vi "BuildPlotsOneGraph.vi"(6 "Legend":string[](array[string]), 7 "Desired Legends":string[](array[string]), 8 "PlotArray":cluster{dbl[], dbl[]}[](array[cluster]), 9 "Plot Legends":string[](array[string]), 10 "Plotstyles":T1[](array[typedef]) {"LineType" min=1 max=6 step=1; "LineWidth" min=1 max=6 step=1; "PointSize" min=0 step=0.1}, 11 "PlotCommand":string) -> (0 "Yspan":dbl, 1 "Xspan":dbl, 3 "String out":string, 4 "Y array":dbl[](array[numeric]), 5 "X array":dbl[](array[numeric]))   [LabVIEW 2012]
uses:
  plotstyle.ctl
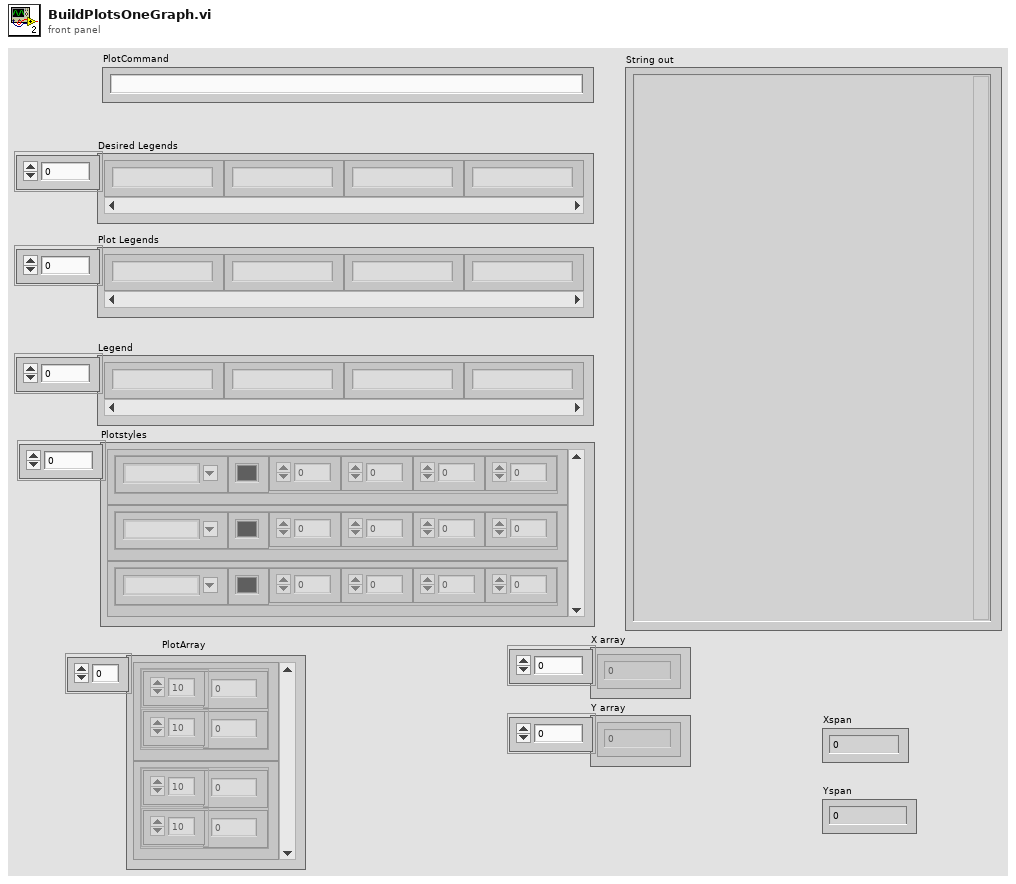
[diagram p1: front panel]
types:
  T1 = typedef "plotstyle.ctl" = cluster{"Style":string, "Color":u32, "PointType":i32, "PointSize":sgl, "LineWidth":sgl, "LineType":u8}
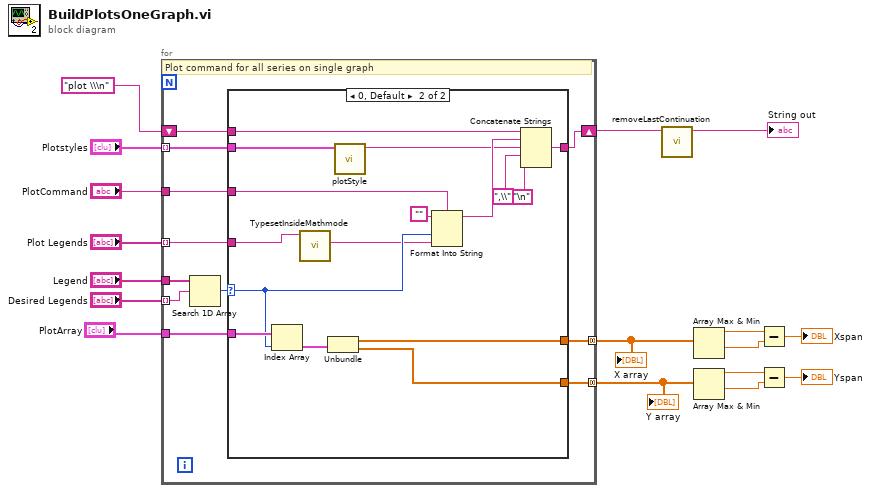
[diagram p0: block diagram]
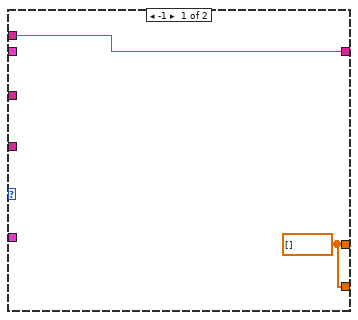
[diagram p2: hidden frame]
diagram:
  n1 = for {
    tunnel: "Plotstyles" -> [w28] mode=indexing
    tunnel: "Plot Legends" -> [w25] mode=indexing
    shift-right: [w26] -> w15
    shift-left: "plot \\\n" -> [w27]
    tunnel: "Desired Legends" -> [w23] mode=indexing
    tunnel: "Legend" -> [w24]
    tunnel: "PlotCommand" -> [w21]
    tunnel: "PlotArray" -> [w20]
    tunnel: [w19] -> w6 mode=concatenating
    tunnel: [w18] -> w3 mode=concatenating
    # "Plot command for all series on single graph"
    n2 = Search 1D Array(1D array=w24, element=w23) -> (index of element=w22:i32)  [unwired: 1 in]
    n3 = case shown="0, Default" w22 {
      selector: w22 -> [_ w36]
      tunnel: w28 -> [_ w45]
      tunnel: w27 -> [w30 w40]
      tunnel: [w30 w39] -> w26
      tunnel: w25 -> [_ w32]
      tunnel: w21 -> [_ w38]
      tunnel: w20 -> [_ w37]
      tunnel: [w29 w34] -> w19
      tunnel: [w29 w33] -> w18
      frame -1 {
        w29 = dbl[] []
      }
      frame 0, Default {
        n4 = Index Array(array=w37, index=w36) -> (element=w35:cluster{dbl[], dbl[]})
        n5 = call "TypesetInsideMathmode.vi"("DirtyString"=w32) -> ("Mathmode String"=w31:string)  [unwired: 9 in, 1 out]
        n6 = Unbundle(w35) -> (w34:dbl[], w33:dbl[])
        n7 = call "plotStyle.vi"("plotSpec"=w45) -> ("String"=w42:string)  [unwired: 10 in]
        n8 = Format Into String(format string=w38, initial string="", w36, w31) -> (resulting string=w43:string)  [unwired: 1 in, 1 out]
        n9 = Concatenate Strings(w40, w43, w42, ",\\" ("string"), "\n") -> (w39:string)
      }
    }
  }
  "X array" <- w6
  "Y array" <- w3
  n10 = call "removeLastContinuation.vi"("String in"=w15) -> ("String out"=→"String out":string)  [unwired: 10 in]
  n11 = Array Max & Min(array=w6) -> (max value=w8:dbl, min value=w7:dbl)  [unwired: 2 out]
  n12 = Array Max & Min(array=w3) -> (max value=w4:dbl, min value=w5:dbl)  [unwired: 2 out]
  n13 = Subtract(x=w8, y=w7) -> (x-y=→"Xspan":dbl)
  n14 = Subtract(x=w4, y=w5) -> (x-y=→"Yspan":dbl)
